vi "Get weather data.vi"() -> (1 "Wather160 data":string[](array[string]))   [LabVIEW 2018]
uses:
  Global_Telescopio.vi
panel:
  # "Temp     Hi      Low     Out    Dew  Wind  Wind   Wind    Hi    Hi   Wind   Heat  THW  THSW             Solar   Solar   Hi Solar   UV    UV      Hi     Heat    Cool    In           In          In       In    Wind  Wind   ISS   Arc.\n  Date    Time     Out   Temp   Temp   Hum    Pt.  Speed   Dir      Run  Speed   Dir  Chill  Index  Index  Index    Bar     Rad.  Energy    Rad.  Index  Dose   UV     D-D     D-D    Temp   Hum    Dew   Heat     ET   Samp   Tx   Recept  Int."
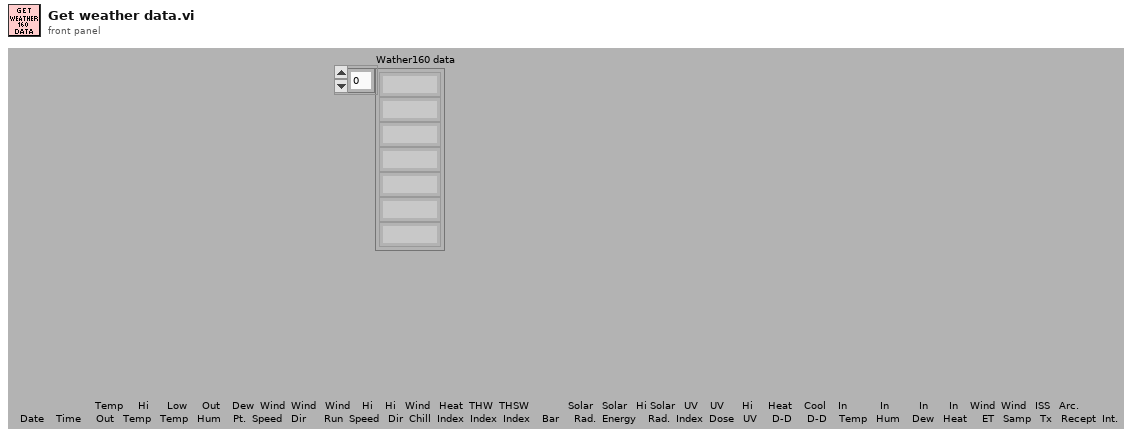
[diagram p1: front panel]
types:
  T1 = cluster{"broker":string, "version":string, "date":string, "hour":string, "outTemp":string, "hiTemp":string, "lowTemp":string, "outHumidity":string, "dewOut":string, "windSpeed":string, "windDirection":string, "windRun":string, "hiSpeed":string, "hiDir":string, "windChill":string, "heatIndex":string, "THWIndex":string, "THSIndex":string, "pressure":string, "rain":string, "rainRate":string, "solarRad":string, "solarEnergy":string, "hiSolarRad":string, "UVIndex":string, "UVDose":string, "hiUV":string, "headDD":string, "coolDD":string, "inTemp":string, "inHumidity":string, "inHeat":string, "inEMC":string, "inAirDensity":string, "2ndTemp":string, "2ndHumidity":string, "ET":string, "leaf":string, "windSamp":string, "windTx":string, "ISSRecept":string, "dewIn":string, "arcInt":string}
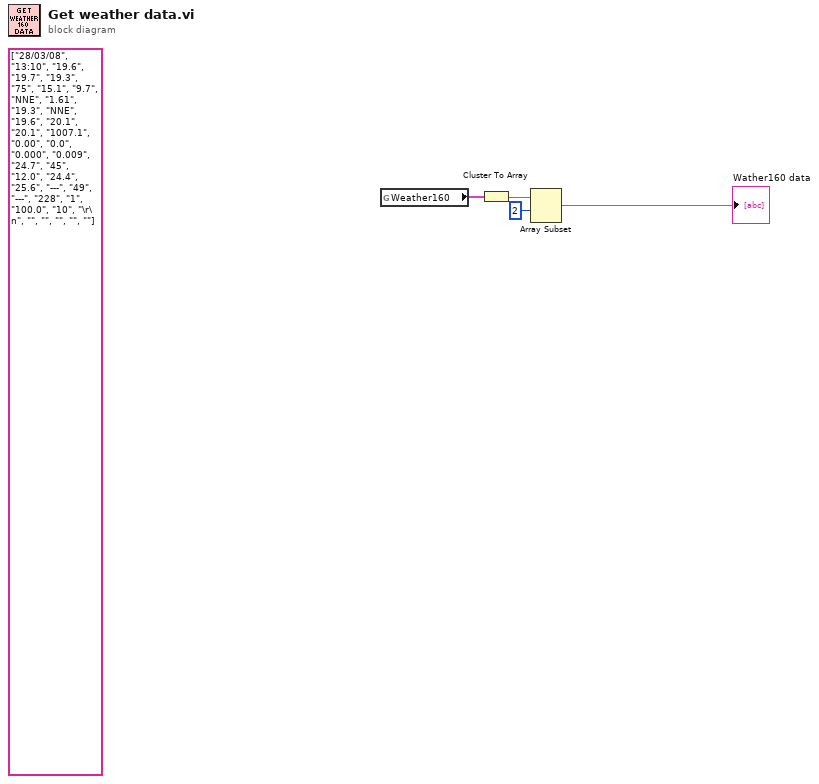
[diagram p0: block diagram]
diagram:
  (unwired) string[] ["28/03/08", "13:10", "19.6", "19.7", "19.3", "75", "15.1", "9.7", "NNE", "1.61", "19.3", "NNE", "19.6", "20.1", "20.1", "1007.1", "0.00", "0.0", "0.000", "0.009", "24.7", "45", "12.0", "24.4", "25.6", "---", "49", "---", "228", "1", "100.0", "10", "\r\n", "", "", "", "", ""] ("Array 2")
  n1 = global read "Global_Telescopio.vi" "Weather160"() -> (w3:T1)
  n2 = Cluster To Array(cluster=w3) -> (array=w4:string[])
  n3 = Array Subset(array=w4, index=2) -> (→"Wather160 data":string[])  [unwired: 1 in]
